vi "LoggerAR_Loop.vi"(8 "error in (no error)":errorcluster) -> (0 "error out":errorcluster)   [LabVIEW 2016]
uses:
  Classes/DataLogger/Data Logger.lvclass
  <vilib>/Platform/TimedLoop/XDataNode/timing_clust.ctl
  <vilib>/Platform/TimedLoop/XDataNode/nitl_modes.ctl
  <vilib>/Platform/TimedLoop/XDataNode/wakeup.ctl
  GlobalVariables/Path_GV.vi
  <vilib>/Platform/TimedLoop/XDataNode/XDataNode.xnode
  <vilib>/Platform/TimedLoop/XDataNode/XDNodeRunTimeDep.lvlib
  <vilib>/GoldZinc Software/auzn custom VIs/CustomVI.lvlib
panel:
  out "Save Time":dbl
  out "ColumnOfVar":i32[](array[numeric])
  out "NumOfColumn":i32
  out "StartTime":dbl
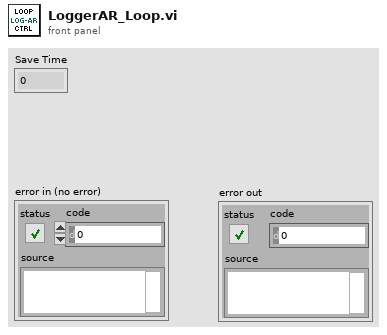
[diagram p1: front panel]
types:
  T1 = enum16{"Idle", "CloseFile", "WriteFile", "CreateFile"}
  T2 = typedef "XDNodeRunTimeDep.lvlib/timing_clust.ctl" = cluster{"Expected End [f-1]":u64, "Actual End [f-1]":u64, "Finished Late? [f-1]":bool, "Expected End [i-1]":u64, "Actual End [i-1]":u64, "Finished Late? [i-1]":bool, "Expected Start [i]":u64, "Actual Start [i]":u64, "Expected Start [f]":u64, "Actual Start [f]":u64, "Source Name":string, "Structure Name":string, "Period":i64, "Deadline":i64, "Offset":i64, "Start":i64, "Priority":i32, "Timeout":i32, "Mode":T3, "Wakeup Reason":T4, "Error":errorcluster, "Source Type":string, "Secondary Source Type":string, "Global End Time":u64, "Global Start Time":u64, "Frame Duration":u64, "Iteration Duration":u64, "Assigned CPU":i32, "I/O Scan Engine Mode":u32}
  T3 = typedef "XDNodeRunTimeDep.lvlib/nitl_modes.ctl" = enum32{"No Change", "Process missed periods, maintain original phase", "Discard missed periods, maintain original phase", "Process missed periods, ignore original phase", "Discard missed periods, ignore original phase"}
  T4 = typedef "XDNodeRunTimeDep.lvlib/wakeup.ctl" = enum32{"Normal", "Aborted", "Asynchronous wakeup", "Timing source error", "Timed loop error", "Timeout"}
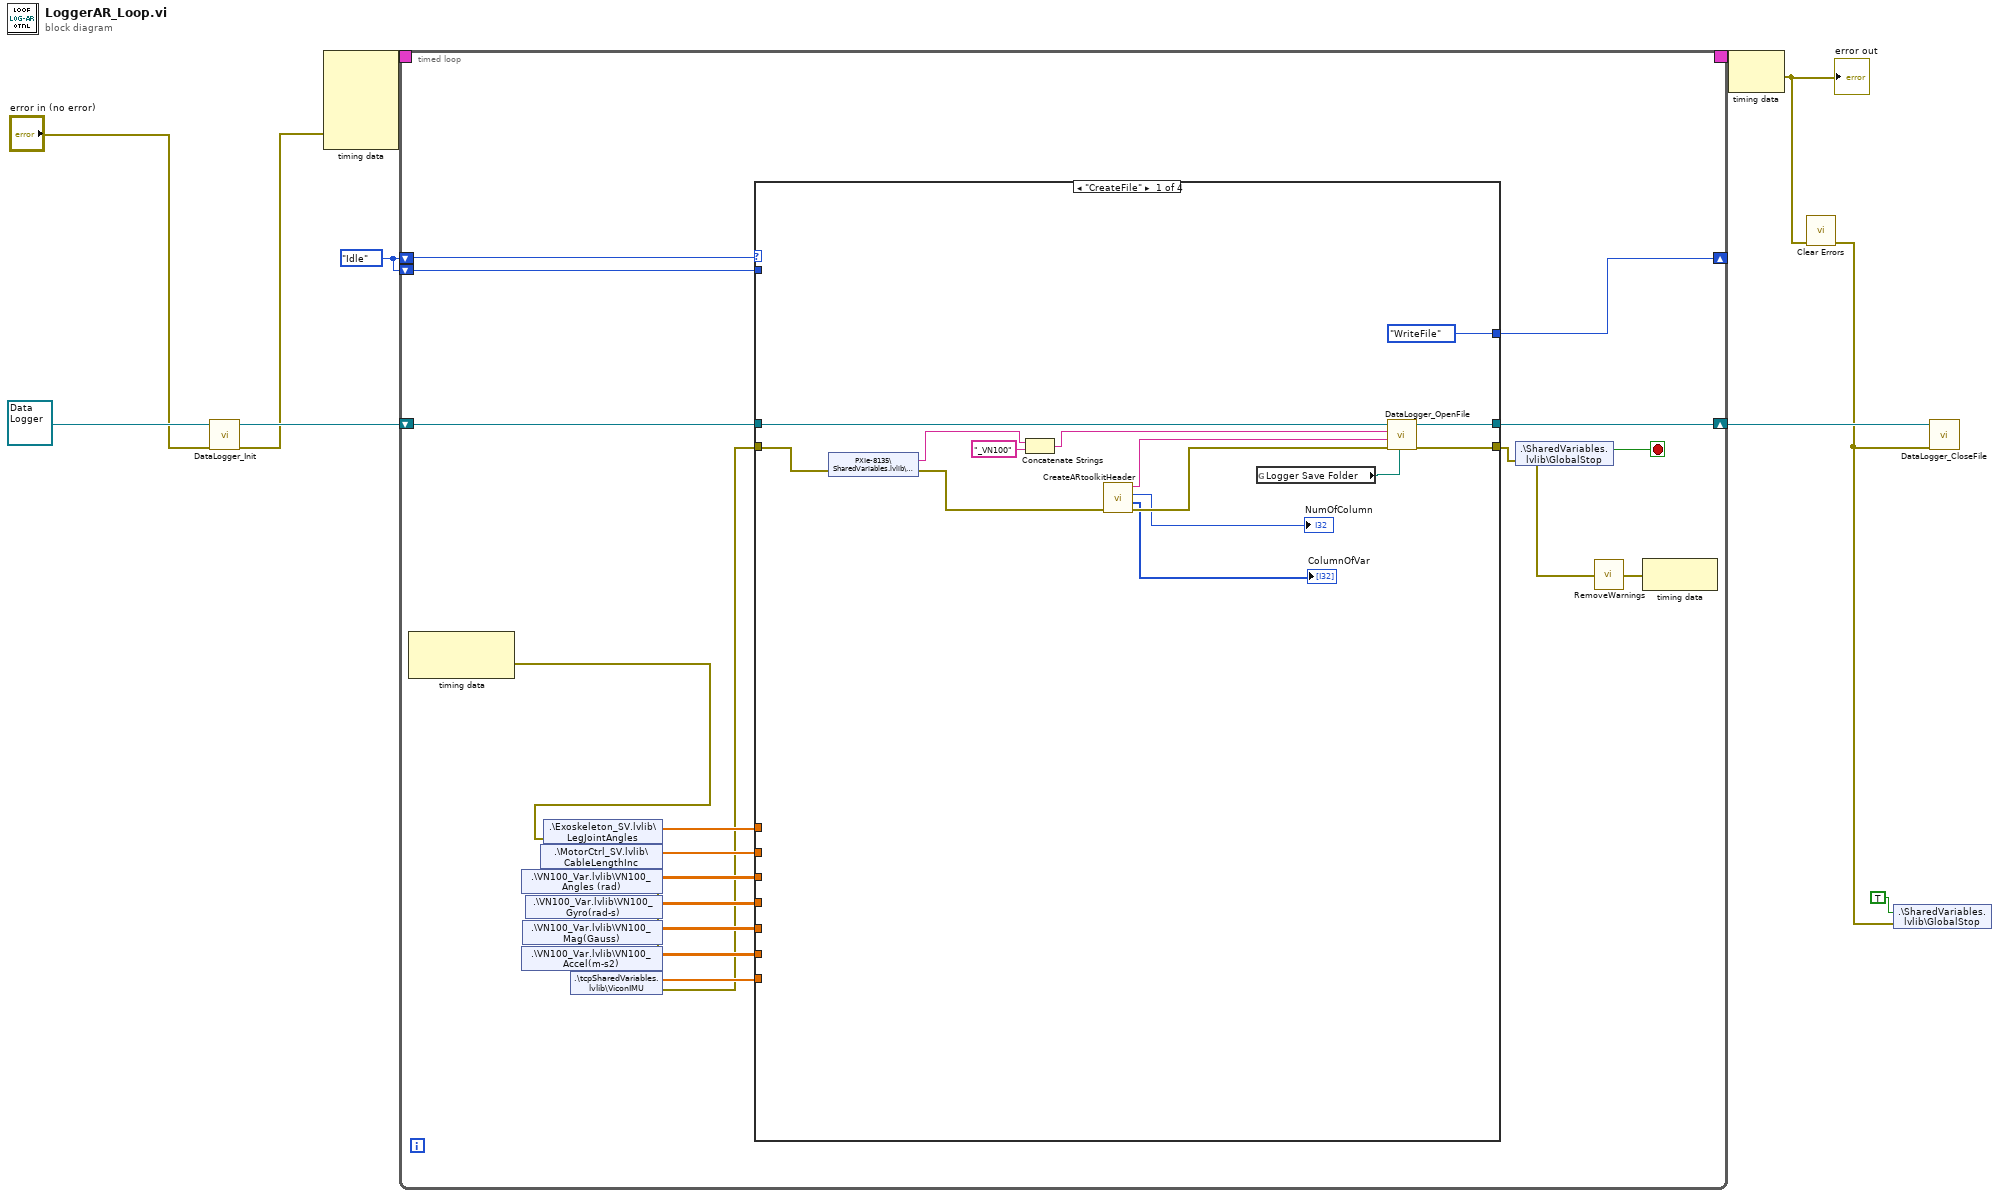
[diagram p0: block diagram]
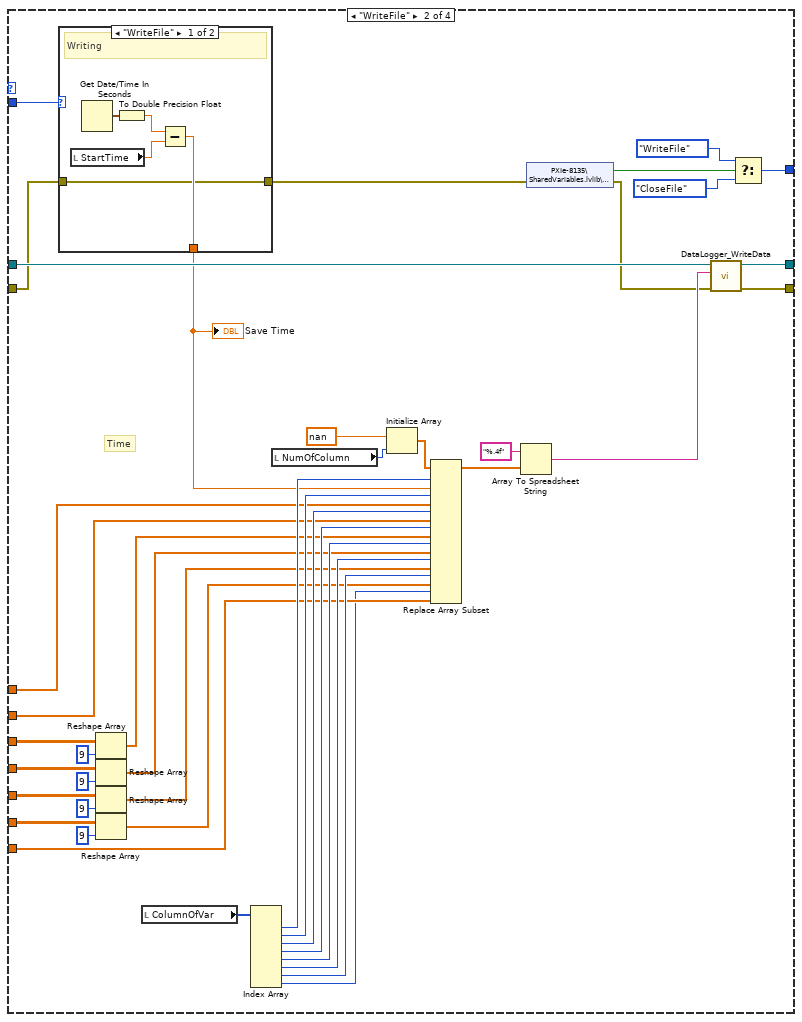
[diagram p2: hidden frame]
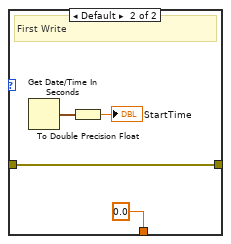
[diagram p3: hidden frame]
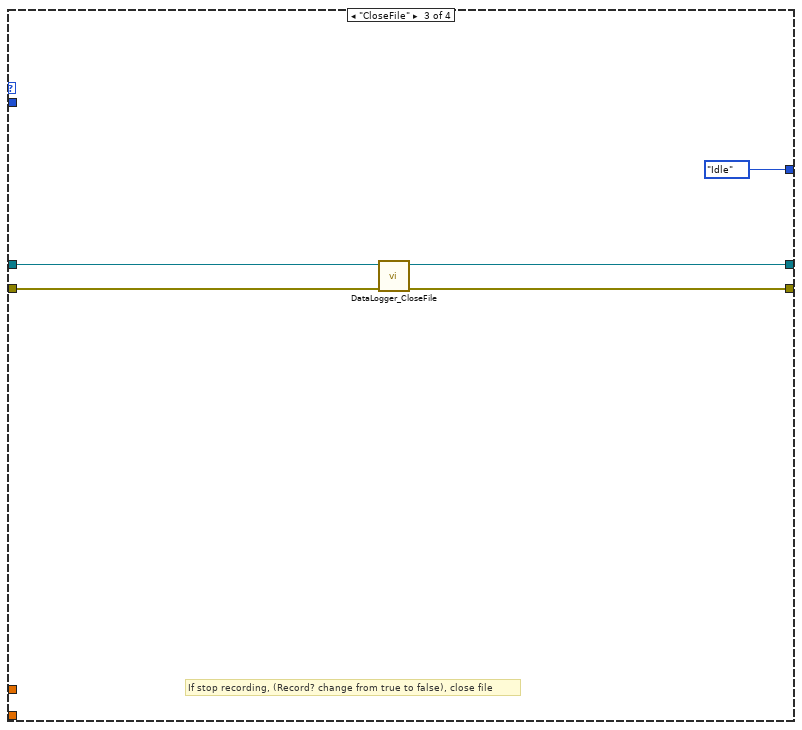
[diagram p4: hidden frame]
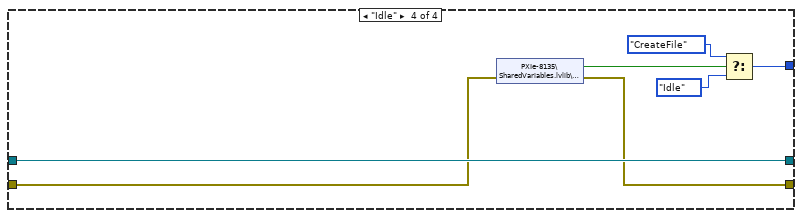
[diagram p5: hidden frame]
diagram:
  w9 = T1."Idle"
  n1 = call "DataLogger_Init.vi"("error in (no error)"="error in (no error)", "Data Logger in"=refnum<class "Data Logger.lvclass"> refnum) -> ("error out"=w1:errorcluster, "Data Logger out"=w3:refnum<class "Data Logger.lvclass">)  [unwired: 8 in]
  n2 = node-c288(w1) -> (w11:T2)  [unwired: 4 in]
  n3 = timed-loop {
    timing: w11 -> [_]
    timing-out: [_] -> w10
    shift-right: [w34] -> w7
    shift-left: w3 -> [w35]
    shift-right: [w33] -> _
    shift-left: w9 -> [w32]
    shift-left: w9 -> [w31]
    stop <- w30 stop-if-true
    n4 = node-c288() -> (w12:errorcluster)  [unwired: 1 in, 1 out]
    n5 = shared-variable ".\\Exoskeleton_SV.lvlib\\LegJointAngles"(error in=w12) -> (w18:dbl[], error out=w16:errorcluster)
    n6 = shared-variable ".\\MotorCtrl_SV.lvlib\\CableLengthInc"(error in=w16) -> (w14:dbl[], error out=w15:errorcluster)
    n7 = shared-variable ".\\VN100_Var.lvlib\\VN100_Angles (rad)"(error in=w15) -> (w25:dbl[][], error out=w28:errorcluster)
    n8 = shared-variable ".\\VN100_Var.lvlib\\VN100_Gyro(rad-s)"(error in=w28) -> (w24:dbl[][], error out=w27:errorcluster)
    n9 = shared-variable ".\\VN100_Var.lvlib\\VN100_Mag(Gauss)"(error in=w27) -> (w23:dbl[][], error out=w26:errorcluster)
    n10 = shared-variable ".\\VN100_Var.lvlib\\VN100_Accel(m-s2)"(error in=w26) -> (w22:dbl[][], error out=w17:errorcluster)
    n11 = shared-variable ".\\tcpSharedVariables.lvlib\\ViconIMU"(error in=w17) -> (w19:dbl[], error out=w13:errorcluster)
    n12 = case shown="\"CreateFile\"" w32 {
      tunnel: w35 -> [w49 w87 w105 w112]
      tunnel: w13 -> [w48 w83 w101 w107]
      tunnel: [w46 w91 w103 w112] -> w34
      tunnel: [w40 w90 w102 w106] -> w29
      tunnel: [T1."WriteFile" w84 T1."Idle" w109] -> w33
      tunnel: w18 -> [_ w60 _ _]
      tunnel: w25 -> [_ w64 _ _]
      tunnel: w24 -> [_ w63 _ _]
      tunnel: w23 -> [_ w62 _ _]
      tunnel: w22 -> [_ w61 _ _]
      tunnel: w31 -> [_ w70 _ _]
      tunnel: w19 -> [_ w55 _ _]
      tunnel: w14 -> [_ w53 _ _]
      frame "CreateFile" {
        n13 = shared-variable "PXIe-8135\\SharedVariables.lvlib\\FileName"(error in=w48) -> (w39:string, error out=w44:errorcluster)
        n14 = Concatenate Strings(w39, "_VN100" ("string")) -> (w38:string)
        n15 = call "CreateARtoolkitHeader.vi"("error in (no error)"=w44) -> ("error out"=w43:errorcluster, "Starting Column of Each Variable"=→"ColumnOfVar":i32[], "Number of Columns"=→"NumOfColumn":i32, "header"=w47:string)  [unwired: 7 in]
        n16 = global read "Path_GV.vi" "Logger Save Folder"() -> (w36:path)
        n17 = call "DataLogger_OpenFile.vi"("base path (C:\\CAlex\\)"=w36, "error in (no error)"=w43, "Header"=w47, "File Name"=w38, "Data Logger in"=w49) -> ("error out"=w40:errorcluster, "Data Logger out"=w46:refnum<class "Data Logger.lvclass">)  [unwired: 5 in]
      }
      frame "WriteFile" {
        # "Time"
        n18 = case shown="\"WriteFile\"" w70 {
          tunnel: w83 -> [w92 w97]
          tunnel: [w92 w97] -> w52
          tunnel: [w93 0.0 ("StartTime")] -> w69
          frame "WriteFile" {
            # "Writing"
            n19 = local read "StartTime"() -> (w94:dbl)
            n20 = Get Date/Time In Seconds() -> (seconds since 1Jan1904=w96:timestamp)
            n21 = To Double Precision Float(number=w96) -> (double precision float=w95:dbl)
            n22 = Subtract(x=w95, y=w94) -> (x-y=w93:dbl)
          }
          frame Default {
            # "First Write"
            n23 = Get Date/Time In Seconds() -> (seconds since 1Jan1904=w100:timestamp)
            n24 = To Double Precision Float(number=w100) -> (double precision float=→"StartTime":dbl)
          }
        }
        "Save Time" <- w69
        n25 = Reshape Array(w64, 9 ("dimension size")) -> (w59:dbl[])
        n26 = Reshape Array(w63, 9 ("dimension size")) -> (w58:dbl[])
        n27 = Reshape Array(w62, 9 ("dimension size")) -> (w57:dbl[])
        n28 = Reshape Array(w61, 9 ("dimension size")) -> (w56:dbl[])
        n29 = local read "ColumnOfVar"() -> (w78:i32[])
        n30 = Index Array(array=w78) -> (element #1=w77:i32, element #2=w76:i32, element #3=w75:i32, element #4=w74:i32, element #5=w73:i32, element #6=w72:i32, element #7=w71:i32, element #8=w54:i32)  [unwired: 8 in]
        n31 = local read "NumOfColumn"() -> (w79:i32)
        n32 = Initialize Array(nan ("element"), w79) -> (w89:dbl[])
        n33 = Replace Array Subset(array=w89, new element #1=w69, index #1=w77, new element #2=w60, index #2=w76, new element #3=w53, index #3=w75, new element #4=w59, index #4=w74, new element #5=w58, index #5=w73, new element #6=w57, index #6=w72, new element #7=w56, index #7=w71, new element #8=w55, index #8=w54) -> (w82:dbl[])
        n34 = Array To Spreadsheet String(array=w82, 3:"%.4f" ("format string")) -> (spreadsheet string=w81:string)  [unwired: 1 in]
        n35 = shared-variable "PXIe-8135\\SharedVariables.lvlib\\Record?"(error in=w52) -> (w50:bool, error out=w51:errorcluster)
        n36 = call "DataLogger_WriteData.vi"("error in (no error)"=w51, "New line"=w81, "Data Logger in"=w87) -> ("error out"=w90:errorcluster, "Data Logger out"=w91:refnum<class "Data Logger.lvclass">)  [unwired: 7 in]
        n37 = Select(t=T1."WriteFile", s=w50, f=T1."CloseFile") -> (s? t:f=w84:T1)
      }
      frame "CloseFile" {
        # "If stop recording, (Record? change from true to false), close file"
        n38 = call "DataLogger_CloseFile.vi"("error in (no error)"=w101, "Data Logger in"=w105) -> ("error out"=w102:errorcluster, "Data Logger out"=w103:refnum<class "Data Logger.lvclass">)  [unwired: 8 in]
      }
      frame "Idle" {
        n39 = shared-variable "PXIe-8135\\SharedVariables.lvlib\\Record?"(error in=w107) -> (w108:bool, error out=w106:errorcluster)
        n40 = Select(t=T1."CreateFile", s=w108, f=T1."Idle") -> (s? t:f=w109:T1)
      }
    }
    n41 = shared-variable ".\\SharedVariables.lvlib\\GlobalStop"(error in=w29) -> (w30:bool, error out=w20:errorcluster)
    n42 = call <vilib>:"RemoveWarnings.vi"("error in (no error)"=w20) -> ("error out"=w21:errorcluster)
    n43 = node-c288(w21) -> ()  [unwired: 1 out]
  }
  n44 = node-c288(w10) -> (w6:errorcluster)
  "error out" <- w6
  n45 = call <vilib>:"Clear Errors.vi"("error in (no error)"=w6) -> ("error out"=w5:errorcluster)  [unwired: 5 in, 1 out]
  n46 = shared-variable ".\\SharedVariables.lvlib\\GlobalStop"(TRUE ("GlobalStop"), error in=w5) -> ()  [unwired: 1 out]
  n47 = call "DataLogger_CloseFile.vi"("error in (no error)"=w5, "Data Logger in"=w7) -> ()  [unwired: 8 in, 2 out]
